vi "pumonarytesting_works_graphing_trial.vi"() -> ()   [LabVIEW 2014]
uses:
  <vilib>/vision/NI_Vision_Development_Module.lvlib
  <instrlib>/KD Scientific 2XX Series/KD Scientific 2XX Series.lvlib
panel:
  in  "Zero Error 2":dbl[](array[numeric])
  in  "Calibration factor 2":dbl[](array[numeric])
  out "Data from Transducer 2":dynamicdata(graph) caption="Voltage from Transducer V"
  in  "stop (F) 2":bool caption="stop (F)"
  in  "Number of Cycles":i32
  in  "Min Pressure":dbl
  in  "Max Pressure":dbl
  out "Status":T1
  in  "stop 2":bool
  out "Delivered Volume":dbl
  out "Units":string
  in  "Baud Rate (9600)":u32(ring)=9600 items=["300"=300, "1200"=1200, "2400"=2400, "4800"=4800, "9600"=9600]
  in  "Withdrawal Settings":T2={"Flow Rate (5)"=5.0, "Volume (10)"=10.0, "Volume Units (ml)"=enum."milliliters (ml)", "Rate Units (ml/min.)"=enum."milliliters per minute (ml/min.)"} {"Volume (10)" format="%#.3g"}
  in  "Diameter (8.75 mm)":dbl=8.75
  in  "Infusion Settings":T2={"Flow Rate (5)"=5.0, "Volume (10)"=10.0, "Volume Units (ml)"=enum."milliliters (ml)", "Rate Units (ml/min.)"=enum."milliliters per minute (ml/min.)"}
  in  "Address (0)":i32 format="%0.0f"
  in  "error in (no error)":errorcluster
  in  "VISA resource name":refnum<visa-resource-name>="COM1"
  in  "stop 4":bool
  in  "stop":bool
  out "Image":T3(plugin-control)
  out "Particle Measurements (Pixels) (Particle Analysis 1)":dbl[][](array[numeric]) format="%.2f"
  out "subarray":dbl[](array[numeric])
  out "The diameter":dbl[](array[numeric])
  in  "stop (F)":bool
  out "Data from Transducer":dynamicdata(graph) caption="Voltage from Transducer V"
  out "Voltage from pressure transducer":dbl[](array[numeric])
  out "Pressure mm Hg":dbl[](graph)
  in  "Calibration factor":dbl[](array[numeric])
  in  "Zero Error":dbl[](array[numeric])
  out "pressure mm Hg":dbl[](array[numeric])
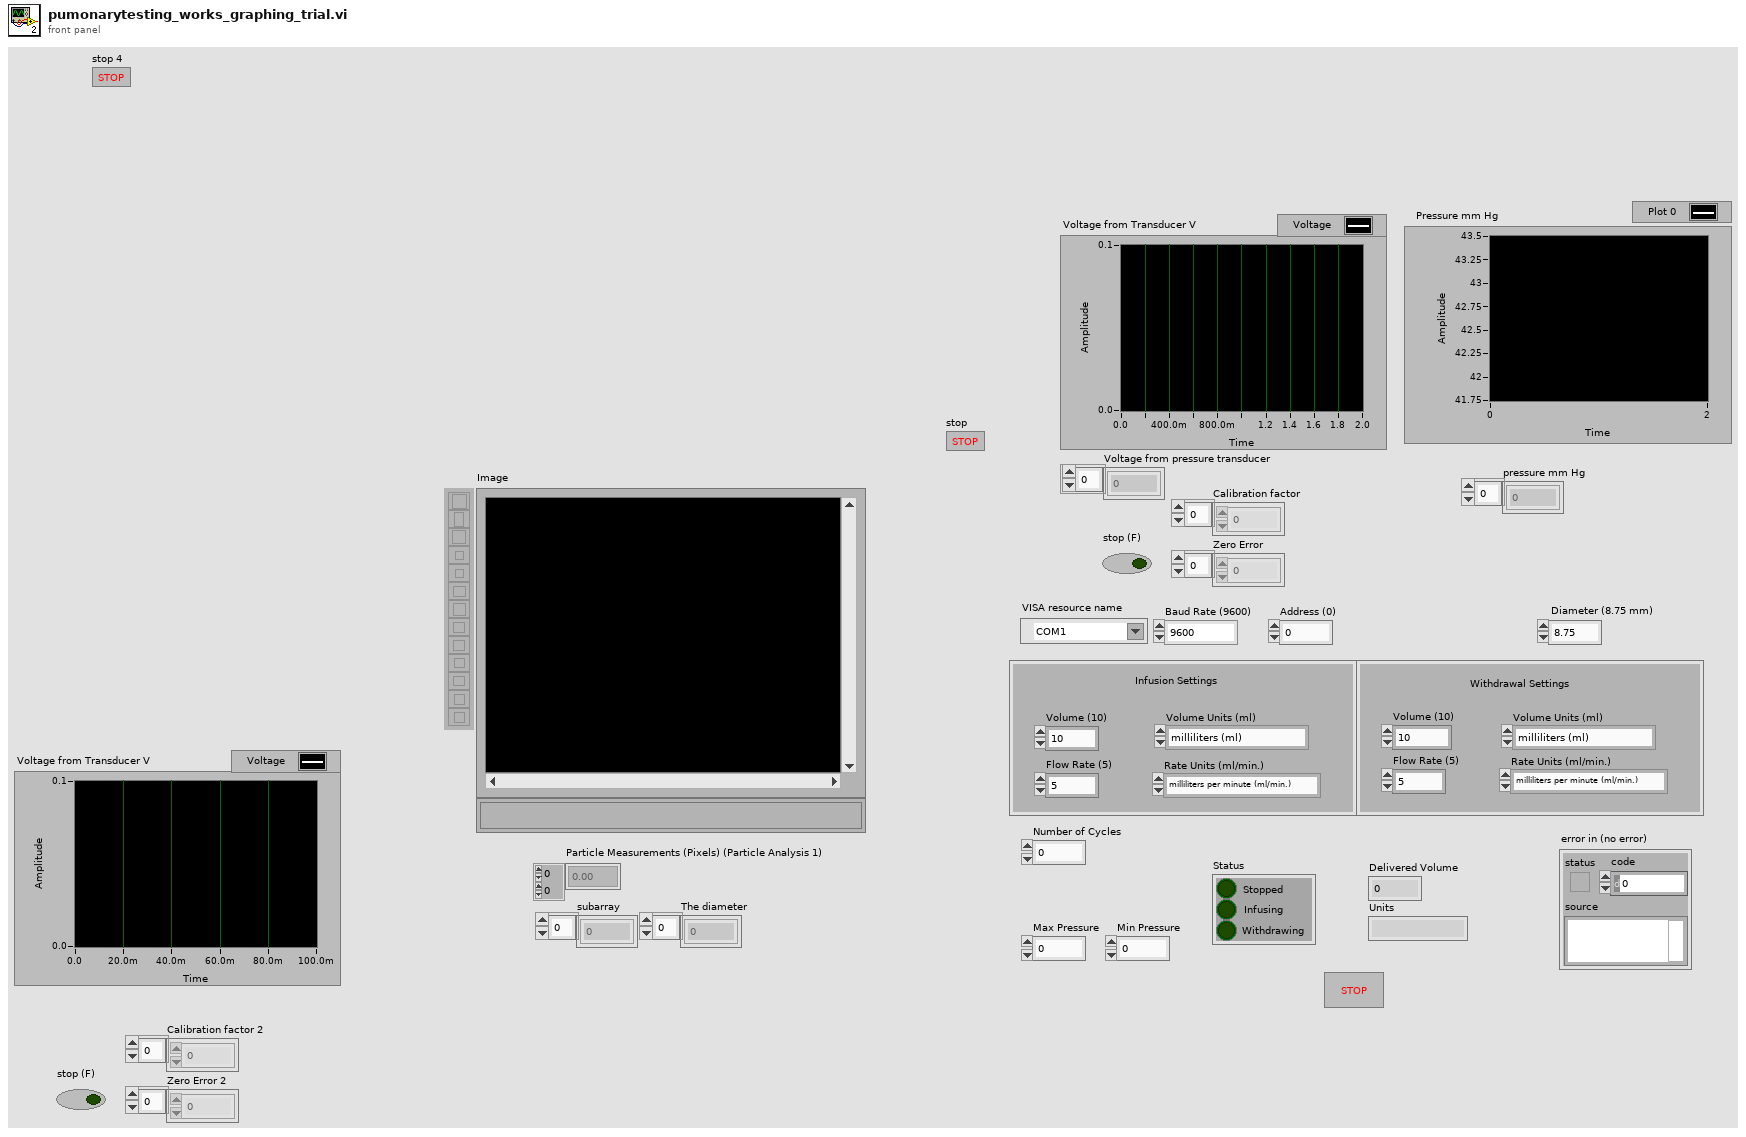
[diagram p1: front panel]
types:
  T1 = cluster{"Stopped":bool, "Infusing":bool, "Withdrawing":bool}
  T2 = cluster{"Flow Rate (5)":dbl, "Volume (10)":dbl, "Volume Units (ml)":enum16{"milliliters (ml)", "microliters (ul)"}, "Rate Units (ml/min.)":enum16{"milliliters per minute (ml/min.)", "milliliters per hour (ml/hr.)", "microliters per minute (ul/min.)", "microliters per hour (ul/hr.)"}}
  T3 = typedef "IMAQ Image.ctl" = refnum<image>
  T4 = typedef "Board Id" = u8
  T5 = typedef "ROI Descriptor" = cluster{"Global Rectangle":i32[], "Contours":cluster{"ID":enum32{"External", "Internal"}, "Type":u32, "Coordinates":i32[]}[]}
  T6 = enum16{"milliliters per minute (ml/min.)", "milliliters per hour (ml/hr.)", "microliters per minute (ul/min.)", "microliters per hour (ul/hr.)"}
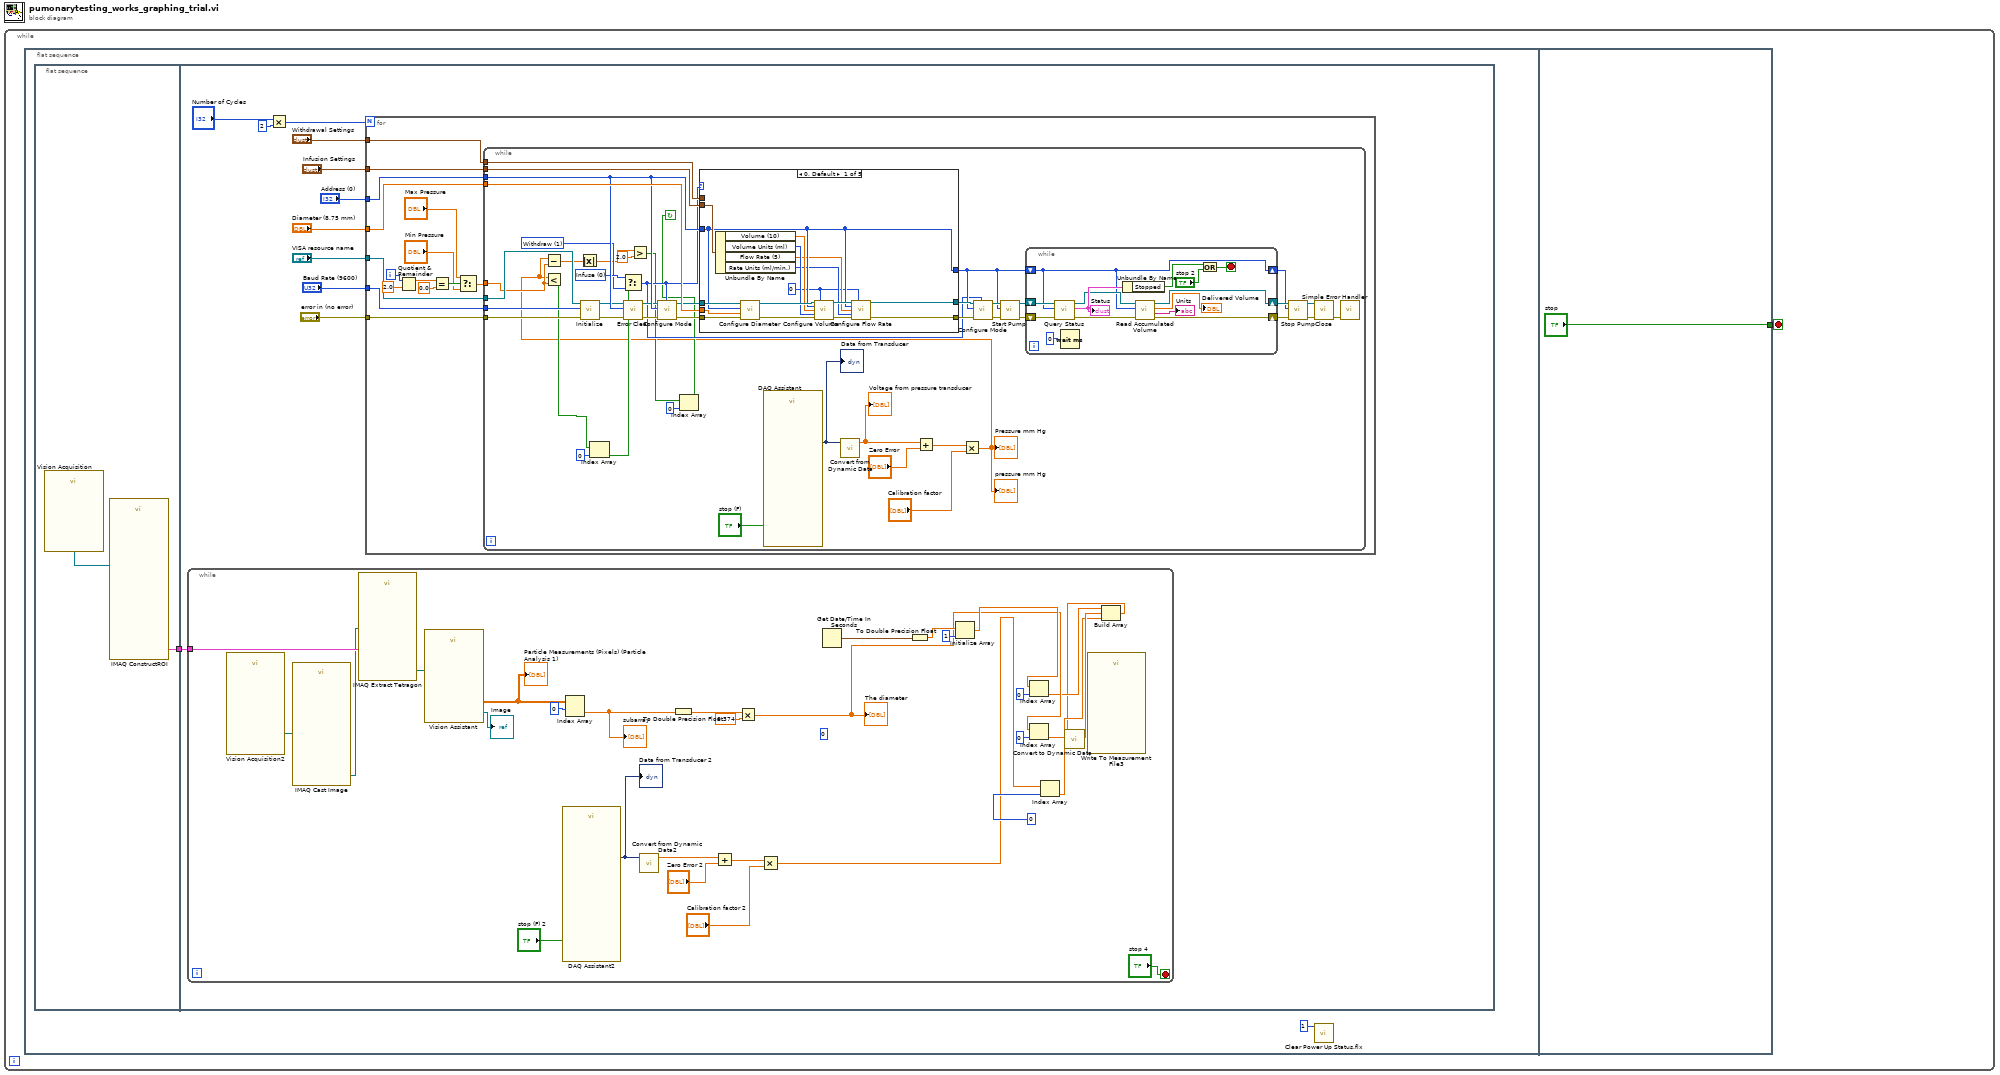
[diagram p0: block diagram]
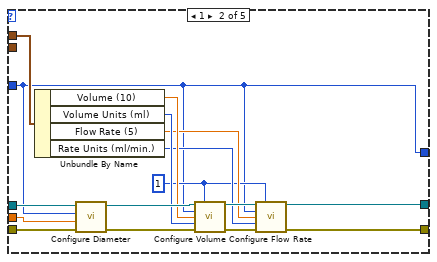
[diagram p2: hidden frame]
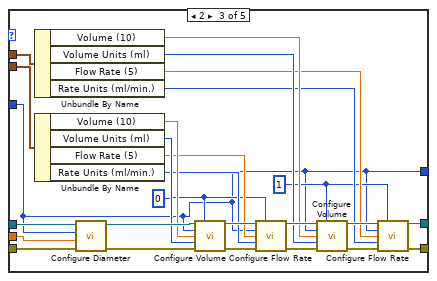
[diagram p3: hidden frame]
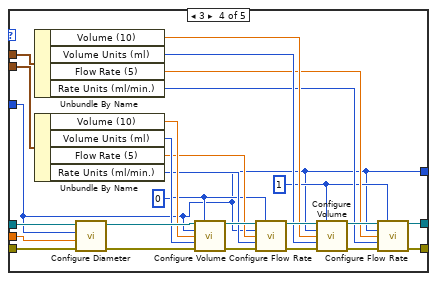
[diagram p4: hidden frame]
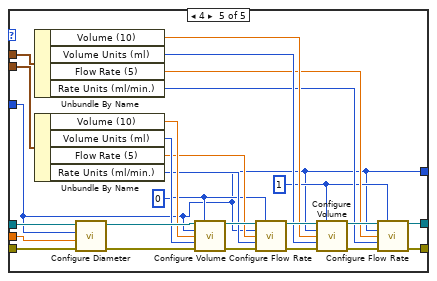
[diagram p5: hidden frame]
diagram:
  n1 = while {
    stop <- w1 stop-if-true
    n2 = flat-sequence {
      tunnel: ["stop"] -> w1
      frame #0 {
        n3 = flat-sequence {
          tunnel: [w4] -> w3
          tunnel: w3 -> [w16]
          frame #0 {
            n4 = call "Vision Acquisition"() -> ("Image Out"=w5:T3)  [unwired: 26 in, 1 out]
            n5 = call "IMAQ ConstructROI"("Image"=w5) -> ("ROI Descriptor Out"=w4:T5)  [unwired: 7 in, 3 out]
          }
          frame #1 {
            n6 = while {
              tunnel: w16 -> [w232]
              stop <- "stop 4" stop-if-true
              (unwired) 0 ("index")
              n7 = call "Vision Acquisition2"() -> ("Image Out"=w223:T3)  [unwired: 25 in, 2 out]
              n8 = call "IMAQ Cast Image"("Image Src"=w223) -> ("Image Dst Out"=w229:T3)  [unwired: 9 in, 1 out]
              n9 = call-poly "IMAQ Extract Tetragon"("ROI Descriptor"=w232, "Image Src"=w229) -> ("Image Dst Out"=w230:T3)  [unwired: 8 in, 1 out]
              n10 = call "Vision Assistant"("Image In"=w230) -> ("Image Out"=→"Image":T3, "Particle Measurements (Pixels) (Particle Analysis 1)"=w228:dbl[][])  [unwired: 23 in, 2 out]
              "Particle Measurements (Pixels) (Particle Analysis 1)" <- w228
              n11 = call "DAQ Assistant2"("stop (F)"="stop (F) 2") -> ("data"=w213:dynamicdata)  [unwired: 15 in, 3 out]
              "Data from Transducer 2" <- w213
              n12 = Index Array(array=w228, index (row)=0) -> (element=w226:dbl[])  [unwired: 1 in]
              "subarray" <- w226
              n13 = call "Convert from Dynamic Data2"("Dynamic Data Type"=w213) -> ("Array"=w216:dbl[])  [unwired: 3 in]
              n14 = To Double Precision Float(number=w226) -> (double precision float=w225:dbl[])
              n15 = Add(x=w216, y="Zero Error 2") -> (x+y=w214:dbl[])
              n16 = Multiply(x=w225, y=0.374) -> (x*y=w208:dbl[])
              "The diameter" <- w208
              n17 = Multiply(x=w214, y="Calibration factor 2") -> (x*y=w207:dbl[])
              n18 = Get Date/Time In Seconds() -> (seconds since 1Jan1904=w221:timestamp)
              n19 = To Double Precision Float(number=w221) -> (double precision float=w220:dbl)
              n20 = Initialize Array(w220, 1 ("dimension size")) -> (w209:dbl[])
              n21 = Index Array(array=w209, index=0) -> (element=w206:dbl)
              n22 = Index Array(array=w208, index=0) -> (element=w205:dbl)
              n23 = Index Array(array=w207, index=0) -> (element=w204:dbl)
              n24 = Build Array(w206, w205, w204) -> (w203:dbl[])
              n25 = call "Convert to Dynamic Data"("Array"=w203) -> ("Dynamic Data Type"=w202:dynamicdata)  [unwired: 3 in]
              n26 = call "Write To Measurement File3"("Signals"=w202) -> ()  [unwired: 16 in, 3 out]
            }
            n27 = Multiply(x="Number of Cycles", y=2) -> (x*y=w15:i32)
            n28 = for {
              N: w15 -> [_]
              tunnel: "VISA resource name" -> [w31]
              tunnel: "error in (no error)" -> [w30]
              tunnel: "Infusion Settings" -> [w29]
              tunnel: "Withdrawal Settings" -> [w28]
              tunnel: "Diameter (8.75 mm)" -> [w27]
              tunnel: "Baud Rate (9600)" -> [w26]
              tunnel: "Address (0)" -> [w25]
              i -> [w23]
              n29 = Quotient & Remainder(x=w23, y=2.0) -> (x-y*floor(x/y)=w21:dbl)  [unwired: 1 out]
              n30 = Equal?(x=w21, y=0.0) -> (x = y?=w20:bool)
              n31 = Select(t="Max Pressure", s=w20, f="Min Pressure") -> (s? t:f=w17:dbl)
              n32 = while {
                tunnel: w31 -> [w77]
                tunnel: w30 -> [w76]
                tunnel: w29 -> [w75]
                tunnel: w28 -> [w74]
                tunnel: w27 -> [w73]
                tunnel: w26 -> [w72]
                tunnel: w25 -> [w71]
                tunnel: w17 -> [w48]
                stop <- w33 continue-if-true
                w50 = u16 1 items=["Withdraw"=1]
                w51 = u16 0 items=["Infuse"] ("Mode (infuse)")
                n33 = call <instrlib>:"Initialize.vi"("error in (no error)"=w76, "Baud Rate (9600)"=w72, "VISA resource name"=w77) -> ("error out"=w53:errorcluster, "VISA resource name out"=w52:refnum<visa-resource-name>)  [unwired: 7 in]
                n34 = call <instrlib>:"Error Clear.vi"("error in (no error)"=w53, "Address (0)"=w71, "VISA resource name"=w52) -> ("error out"=w54:errorcluster, "VISA resource name out"=w55:refnum<visa-resource-name>)  [unwired: 6 in, 1 out]
                n35 = call "DAQ Assistant"("stop (F)"="stop (F)") -> ("data"=w39:dynamicdata)  [unwired: 15 in, 3 out]
                "Data from Transducer" <- w39
                n36 = call "Convert from Dynamic Data"("Dynamic Data Type"=w39) -> ("Array"=w42:dbl[])  [unwired: 3 in]
                "Voltage from pressure transducer" <- w42
                n37 = Add(x=w42, y="Zero Error") -> (x+y=w40:dbl[])
                n38 = Multiply(x=w40, y="Calibration factor") -> (x*y=w32:dbl[])
                "Pressure mm Hg" <- w32
                "pressure mm Hg" <- w32
                n39 = Subtract(x=w32, y=w48) -> (x-y=w47:dbl[])
                n40 = Less?(x=w32, y=w48) -> (x < y?=w38:bool[])
                n41 = Absolute Value(x=w47) -> (abs(x)=w46:dbl[])
                n42 = Index Array(array=w38, index=0) -> (element=w36:bool)
                n43 = Select(t=w51, s=w36, f=w50) -> (s? t:f=w49:u16)
                n44 = Greater?(x=w46, y=2.0) -> (0:w35:bool[])
                n45 = call <instrlib>:"Configure Mode.vi"("Mode (infuse)"=w49, "error in (no error)"=w54, "Address (0)"=w71, "VISA resource name"=w55) -> ("error out"=w57:errorcluster, "VISA resource name out"=w56:refnum<visa-resource-name>)  [unwired: 6 in]
                n46 = Index Array(array=w35, index=0) -> (element=w33:bool)
                n47 = case shown="0, Default" w49 {
                  tunnel: w75 -> [w87 _ w135 w161 w187]
                  tunnel: w74 -> [_ w109 w134 w160 w186]
                  tunnel: w56 -> [w93 w108 w133 w159 w185]
                  tunnel: w57 -> [w92 w104 w132 w158 w184]
                  tunnel: w73 -> [w86 w100 w115 w141 w167]
                  tunnel: [w85 w94 w110 w136 w162] -> w58
                  tunnel: w71 -> [w85 w94 w110 w136 w162]
                  tunnel: [w80 w105 w112 w138 w164] -> w62
                  tunnel: [w79 w101 w111 w137 w163] -> w61
                  frame 0, Default {
                    w78 = 0
                    n48 = Unbundle By Name(w87) -> ("Volume (10)"=w84:dbl, "Volume Units (ml)"=w83:enum16{"milliliters (ml)", "microliters (ul)"}, "Flow Rate (5)"=w82:dbl, "Rate Units (ml/min.)"=w81:T6)
                    n49 = call <instrlib>:"Configure Diameter.vi"("error in (no error)"=w92, "Diameter (8.75 mm)"=w86, "Address (0)"=w85, "VISA resource name"=w93) -> ("error out"=w90:errorcluster, "VISA resource name out"=w91:refnum<visa-resource-name>)  [unwired: 6 in]
                    n50 = call <instrlib>:"Configure Volume.vi"("VISA resource name"=w91, "Mode (infuse)"=w78, "Address (0)"=w85, "Volume (100)"=w84, "Units (0: milliliters)"=w83, "error in (no error)"=w90) -> ("VISA resource name out"=w89:refnum<visa-resource-name>, "error out"=w88:errorcluster)  [unwired: 8 in]
                    n51 = call <instrlib>:"Configure Flow Rate.vi"("VISA resource name"=w89, "Mode (infuse)"=w78, "Address (0)"=w85, "Flow Rate (5)"=w82, "Units (0: milliliters per minute)"=w81, "error in (no error)"=w88) -> ("VISA resource name out"=w80:refnum<visa-resource-name>, "error out"=w79:errorcluster)  [unwired: 8 in]
                  }
                  frame 1 {
                    w95 = 1
                    n52 = Unbundle By Name(w109) -> ("Volume (10)"=w99:dbl, "Volume Units (ml)"=w98:enum16{"milliliters (ml)", "microliters (ul)"}, "Flow Rate (5)"=w97:dbl, "Rate Units (ml/min.)"=w96:T6)
                    n53 = call <instrlib>:"Configure Diameter.vi"("error in (no error)"=w104, "Diameter (8.75 mm)"=w100, "Address (0)"=w94, "VISA resource name"=w108) -> ("error out"=w103:errorcluster, "VISA resource name out"=w107:refnum<visa-resource-name>)  [unwired: 6 in]
                    n54 = call <instrlib>:"Configure Volume.vi"("VISA resource name"=w107, "Mode (infuse)"=w95, "Address (0)"=w94, "Volume (100)"=w99, "Units (0: milliliters)"=w98, "error in (no error)"=w103) -> ("VISA resource name out"=w106:refnum<visa-resource-name>, "error out"=w102:errorcluster)  [unwired: 8 in]
                    n55 = call <instrlib>:"Configure Flow Rate.vi"("VISA resource name"=w106, "Mode (infuse)"=w95, "Address (0)"=w94, "Flow Rate (5)"=w97, "Units (0: milliliters per minute)"=w96, "error in (no error)"=w102) -> ("VISA resource name out"=w105:refnum<visa-resource-name>, "error out"=w101:errorcluster)  [unwired: 8 in]
                  }
                  frame 2 {
                    w113 = 1
                    w114 = 0
                    n56 = Unbundle By Name(w134) -> ("Volume (10)"=w119:dbl, "Volume Units (ml)"=w118:enum16{"milliliters (ml)", "microliters (ul)"}, "Flow Rate (5)"=w117:dbl, "Rate Units (ml/min.)"=w116:T6)
                    n57 = Unbundle By Name(w135) -> ("Volume (10)"=w123:dbl, "Volume Units (ml)"=w122:enum16{"milliliters (ml)", "microliters (ul)"}, "Flow Rate (5)"=w121:dbl, "Rate Units (ml/min.)"=w120:T6)
                    n58 = call <instrlib>:"Configure Diameter.vi"("error in (no error)"=w132, "Diameter (8.75 mm)"=w115, "Address (0)"=w110, "VISA resource name"=w133) -> ("error out"=w127:errorcluster, "VISA resource name out"=w131:refnum<visa-resource-name>)  [unwired: 6 in]
                    n59 = call <instrlib>:"Configure Volume.vi"("VISA resource name"=w131, "Mode (infuse)"=w114, "Address (0)"=w110, "Volume (100)"=w123, "Units (0: milliliters)"=w122, "error in (no error)"=w127) -> ("VISA resource name out"=w130:refnum<visa-resource-name>, "error out"=w126:errorcluster)  [unwired: 8 in]
                    n60 = call <instrlib>:"Configure Flow Rate.vi"("VISA resource name"=w130, "Mode (infuse)"=w114, "Address (0)"=w110, "Flow Rate (5)"=w121, "Units (0: milliliters per minute)"=w120, "error in (no error)"=w126) -> ("VISA resource name out"=w129:refnum<visa-resource-name>, "error out"=w125:errorcluster)  [unwired: 8 in]
                    n61 = call <instrlib>:"Configure Volume.vi"("VISA resource name"=w129, "Mode (infuse)"=w113, "Address (0)"=w110, "Volume (100)"=w119, "Units (0: milliliters)"=w118, "error in (no error)"=w125) -> ("VISA resource name out"=w128:refnum<visa-resource-name>, "error out"=w124:errorcluster)  [unwired: 8 in]
                    n62 = call <instrlib>:"Configure Flow Rate.vi"("VISA resource name"=w128, "Mode (infuse)"=w113, "Address (0)"=w110, "Flow Rate (5)"=w117, "Units (0: milliliters per minute)"=w116, "error in (no error)"=w124) -> ("VISA resource name out"=w112:refnum<visa-resource-name>, "error out"=w111:errorcluster)  [unwired: 8 in]
                  }
                  frame 3 {
                    w139 = 1
                    w140 = 0
                    n63 = Unbundle By Name(w160) -> ("Volume (10)"=w145:dbl, "Volume Units (ml)"=w144:enum16{"milliliters (ml)", "microliters (ul)"}, "Flow Rate (5)"=w143:dbl, "Rate Units (ml/min.)"=w142:T6)
                    n64 = Unbundle By Name(w161) -> ("Volume (10)"=w149:dbl, "Volume Units (ml)"=w148:enum16{"milliliters (ml)", "microliters (ul)"}, "Flow Rate (5)"=w147:dbl, "Rate Units (ml/min.)"=w146:T6)
                    n65 = call <instrlib>:"Configure Diameter.vi"("error in (no error)"=w158, "Diameter (8.75 mm)"=w141, "Address (0)"=w136, "VISA resource name"=w159) -> ("error out"=w153:errorcluster, "VISA resource name out"=w157:refnum<visa-resource-name>)  [unwired: 6 in]
                    n66 = call <instrlib>:"Configure Volume.vi"("VISA resource name"=w157, "Mode (infuse)"=w140, "Address (0)"=w136, "Volume (100)"=w149, "Units (0: milliliters)"=w148, "error in (no error)"=w153) -> ("VISA resource name out"=w156:refnum<visa-resource-name>, "error out"=w152:errorcluster)  [unwired: 8 in]
                    n67 = call <instrlib>:"Configure Flow Rate.vi"("VISA resource name"=w156, "Mode (infuse)"=w140, "Address (0)"=w136, "Flow Rate (5)"=w147, "Units (0: milliliters per minute)"=w146, "error in (no error)"=w152) -> ("VISA resource name out"=w155:refnum<visa-resource-name>, "error out"=w151:errorcluster)  [unwired: 8 in]
                    n68 = call <instrlib>:"Configure Volume.vi"("VISA resource name"=w155, "Mode (infuse)"=w139, "Address (0)"=w136, "Volume (100)"=w145, "Units (0: milliliters)"=w144, "error in (no error)"=w151) -> ("VISA resource name out"=w154:refnum<visa-resource-name>, "error out"=w150:errorcluster)  [unwired: 8 in]
                    n69 = call <instrlib>:"Configure Flow Rate.vi"("VISA resource name"=w154, "Mode (infuse)"=w139, "Address (0)"=w136, "Flow Rate (5)"=w143, "Units (0: milliliters per minute)"=w142, "error in (no error)"=w150) -> ("VISA resource name out"=w138:refnum<visa-resource-name>, "error out"=w137:errorcluster)  [unwired: 8 in]
                  }
                  frame 4 {
                    w165 = 1
                    w166 = 0
                    n70 = Unbundle By Name(w186) -> ("Volume (10)"=w171:dbl, "Volume Units (ml)"=w170:enum16{"milliliters (ml)", "microliters (ul)"}, "Flow Rate (5)"=w169:dbl, "Rate Units (ml/min.)"=w168:T6)
                    n71 = Unbundle By Name(w187) -> ("Volume (10)"=w175:dbl, "Volume Units (ml)"=w174:enum16{"milliliters (ml)", "microliters (ul)"}, "Flow Rate (5)"=w173:dbl, "Rate Units (ml/min.)"=w172:T6)
                    n72 = call <instrlib>:"Configure Diameter.vi"("error in (no error)"=w184, "Diameter (8.75 mm)"=w167, "Address (0)"=w162, "VISA resource name"=w185) -> ("error out"=w179:errorcluster, "VISA resource name out"=w183:refnum<visa-resource-name>)  [unwired: 6 in]
                    n73 = call <instrlib>:"Configure Volume.vi"("VISA resource name"=w183, "Mode (infuse)"=w166, "Address (0)"=w162, "Volume (100)"=w175, "Units (0: milliliters)"=w174, "error in (no error)"=w179) -> ("VISA resource name out"=w182:refnum<visa-resource-name>, "error out"=w178:errorcluster)  [unwired: 8 in]
                    n74 = call <instrlib>:"Configure Flow Rate.vi"("VISA resource name"=w182, "Mode (infuse)"=w166, "Address (0)"=w162, "Flow Rate (5)"=w173, "Units (0: milliliters per minute)"=w172, "error in (no error)"=w178) -> ("VISA resource name out"=w181:refnum<visa-resource-name>, "error out"=w177:errorcluster)  [unwired: 8 in]
                    n75 = call <instrlib>:"Configure Volume.vi"("VISA resource name"=w181, "Mode (infuse)"=w165, "Address (0)"=w162, "Volume (100)"=w171, "Units (0: milliliters)"=w170, "error in (no error)"=w177) -> ("VISA resource name out"=w180:refnum<visa-resource-name>, "error out"=w176:errorcluster)  [unwired: 8 in]
                    n76 = call <instrlib>:"Configure Flow Rate.vi"("VISA resource name"=w180, "Mode (infuse)"=w165, "Address (0)"=w162, "Flow Rate (5)"=w169, "Units (0: milliliters per minute)"=w168, "error in (no error)"=w176) -> ("VISA resource name out"=w164:refnum<visa-resource-name>, "error out"=w163:errorcluster)  [unwired: 8 in]
                  }
                }
                n77 = call <instrlib>:"Configure Mode.vi"("Mode (infuse)"=w49, "error in (no error)"=w61, "Address (0)"=w58, "VISA resource name"=w62) -> ("error out"=w59:errorcluster, "VISA resource name out"=w60:refnum<visa-resource-name>)  [unwired: 6 in]
                n78 = call <instrlib>:"Start Pump.vi"("error in (no error)"=w59, "Address (0)"=w58, "VISA resource name"=w60) -> ("error out"=w69:errorcluster, "VISA resource name out"=w70:refnum<visa-resource-name>)  [unwired: 7 in]
                n79 = while {
                  shift-right: [w190] -> w66
                  shift-left: w58 -> [w190]
                  shift-right: [w192] -> w68
                  shift-left: w70 -> [w198]
                  shift-right: [w191] -> w67
                  shift-left: w69 -> [w199]
                  stop <- w196 stop-if-true
                  n80 = call <instrlib>:"Query Status.vi"("error in (no error)"=w199, "Address (0)"=w190, "VISA resource name"=w198) -> ("error out"=w201:errorcluster, "Status"=w197:T1, "VISA resource name out"=w193:refnum<visa-resource-name>)  [unwired: 6 in]
                  "Status" <- w197
                  n81 = Wait (ms)(milliseconds to wait=u32 0) -> ()  [unwired: 1 out]
                  n82 = Unbundle By Name(w197) -> ("Stopped"=w195:bool)
                  n83 = call <instrlib>:"Read Accumulated Volume.vi"("error in (no error)"=w201, "Address (0)"=w190, "VISA resource name"=w193) -> ("error out"=w191:errorcluster, "Units"=→"Units":string, "Delivered Volume"=→"Delivered Volume":dbl, "VISA resource name out"=w192:refnum<visa-resource-name>)  [unwired: 5 in]
                  n84 = Or(x=w195, y="stop 2") -> (x .or. y?=w196:bool)
                }
                n85 = call <instrlib>:"Stop Pump.vi"("error in (no error)"=w67, "Address (0)"=w66, "VISA resource name"=w68) -> ("error out"=w64:errorcluster, "VISA resource name out"=w63:refnum<visa-resource-name>)  [unwired: 7 in]
                n86 = call <instrlib>:"Close.vi"("error in (no error)"=w64, "VISA resource name"=w63) -> ("error out"=w65:errorcluster)  [unwired: 9 in]
                n87 = call <vilib>:"Simple Error Handler.vi"("error in (no error)"=w65) -> ()  [unwired: 4 in, 5 out]
              }
            }
          }
        }
        n88 = call <vilib>:"Clear Power Up Status.flx"("Board ID"=T4 1) -> ()  [unwired: 6 in, 2 out]
      }
      frame #1 {
      }
    }
  }
